vi "Morlet.vi"(2 "z":dbl[](array[numeric]), 3 "T":dbl[](array[numeric])) -> (0 "dY":dbl[](array[numeric]), 1 "Y":dbl[](array[numeric]))   [LabVIEW 2022 SP3]
uses:
  <vilib>/express/express arith-compare/Formula/XNode/ExpressFormulaBlockNode.xnode
panel:
  in  "W0":dbl
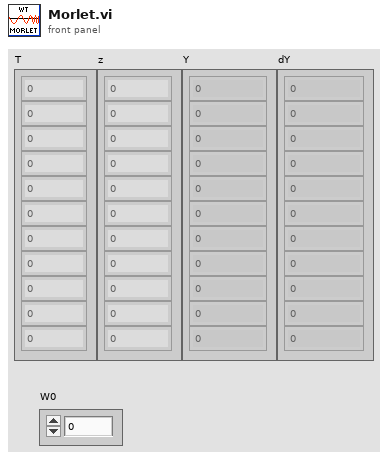
[diagram p1: front panel]
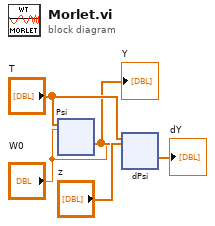
[diagram p0: block diagram]
diagram:
  n1 = xnode "Psi"("t"="T", "w"="W0") -> ("Result"=w2:dbl[])  [unwired: 1 in, 1 out]
  "Y" <- w2
  n2 = xnode "dPsi"("t"="T", "a"="z", "f"=w2, "w"="W0") -> ("Result"=→"dY":dbl[])  [unwired: 1 in, 1 out]
